vi "Enum to All Items.vi"() -> ()   [LabVIEW 2020]
uses:
  Path Control/Paths.ctl
  Path Control/PathControl.lvclass
panel:
  out "Array":string[](array[string])
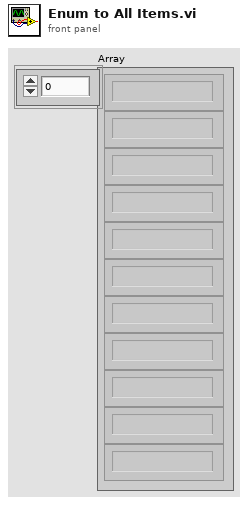
[diagram p1: front panel]
types:
  T1 = typedef "PathControl.lvclass/Paths.ctl" = enum16{"SigGen 1 -> DUT", "SigGen 2 -> DUT", "SigGen 1 -> PM 1", "SigGen 1 -> PM 2", "DUT -> SA", "DUT -> PM 2", "VSG -> DUT", "SigGen 2 -> PM 1", "SigGen 2 -> PM 2"}
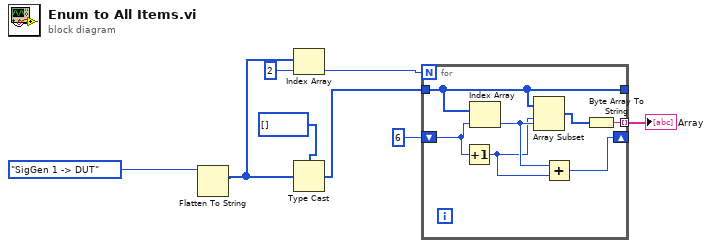
[diagram p0: block diagram]
diagram:
  n1 = Flatten To String(anything=Paths."SigGen 1 -> DUT" ("Path")) -> (type string=w1:i16[])  [unwired: 3 in, 2 out]
  n2 = Index Array(array=w1, index=2) -> (element=w6:i16)
  n3 = Type Cast(type=u8[] [], x=w1) -> (*(type *) &x=w4:u8[])
  n4 = for {
    N: w6 -> [_]
    shift-right: [w11] -> _
    shift-left: 6 -> [w15]
    tunnel: w4 -> [w14]
    tunnel: [w14] -> _
    tunnel: [w9] -> w2 mode=indexing
    n5 = Increment(x=w15) -> (x+1=w12:i32)
    n6 = Index Array(array=w14, index=w15) -> (element=w13:u8)
    n7 = Array Subset(array=w14, index=w12, length=w13) -> (w10:u8[])
    n8 = Add(x=w13, y=w12) -> (x+y=w11:i32)
    n9 = Byte Array To String(unsigned byte array=w10) -> (string=w9:string)
  }
  "Array" <- w2
